vi "Edit Menu (Sub VI).vi"(8 "error in (no error)":errorcluster, 10 "Add/remove":string[](array[string])=["Current", "Temperature", "Voltage"]) -> (0 "error out":errorcluster, 2 "Add/remove 2":string[](array[string])=["Current", "Temperature", "Voltage"])   [LabVIEW 2012]
doc: "This VI allows you to modify the elements in the menu"
panel:
  in  "stop":bool
  # "Instructions:\n1. To delete an element, simply right-click the field and choose Delete Element.\n2. To add an element, right-click the the menu and choose Insert Element before.\n3. Click on OK"
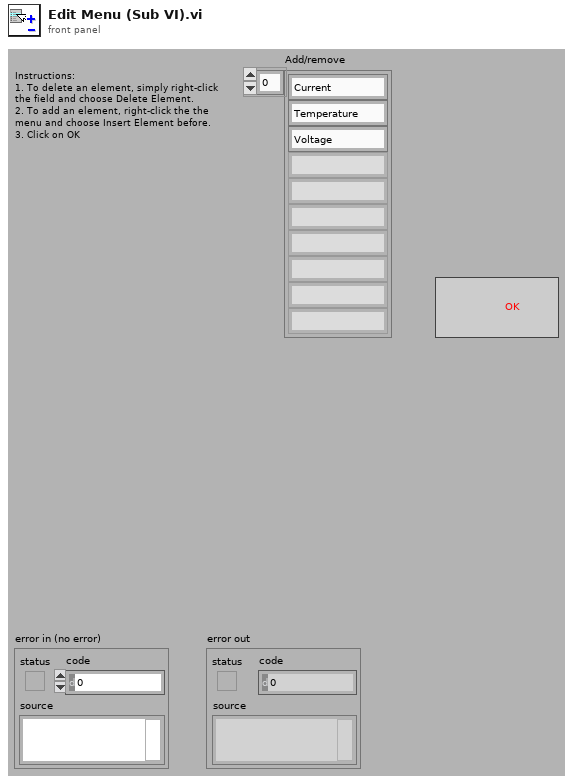
[diagram p1: front panel]
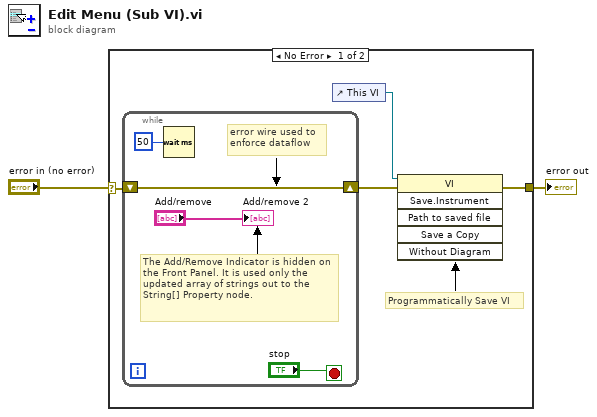
[diagram p0: block diagram]
diagram:
  n1 = case shown="No Error" "error in (no error)" {
    selector: "error in (no error)" -> [w3 w11]
    tunnel: [w4 w11] -> w2
    frame No Error {
      # "Programmatically Save VI"
      n2 = while {
        shift-right: [w7] -> w5
        shift-left: w3 -> [w7]
        stop <- "stop" stop-if-true
        # "error wire used to \nenforce dataflow"
        # "The Add/Remove Indicator is hidden on the Front Panel. It is used only the updated array of strings out to the String[] Property node."
        n3 = Wait (ms)(milliseconds to wait=u32 50) -> ()  [unwired: 1 out]
        "Add/remove 2" <- "Add/remove"
      }
      n4 = control-ref of="This VI"() -> (w6:refnum<vi>)
      n5 = invoke class="VI" method="Save.Instrument"(reference=w6, error in=w5) -> (error out=w4:errorcluster)  [unwired: 4 in, 5 out]
    }
    frame Error {
    }
  }
  "error out" <- w2
